vi "Preview HVAC.vi"(8 "error in (no error)":errorcluster, 11 "HVAC System Model in":refnum<class "HVAC System Model.lvclass">) -> (0 "error out":errorcluster, 3 "HVAC System Model out":refnum<class "HVAC System Model.lvclass">)   [LabVIEW 2013, in "HVAC System Model.lvlib" / "HVAC System Model.lvclass"]
uses:
  HVAC System Model.lvclass
  HVAC System Model.lvclass/HVAC System Model.ctl
  <vilib>/xml/Load XML File.vi
  <vilib>/xml/Close Reference(Node).vi
  Common/File IO/File IO.lvlib
  <vilib>/xml/NI_XML.lvlib
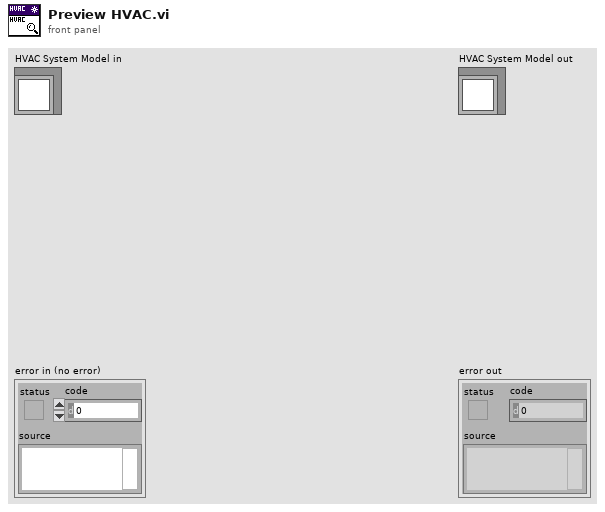
[diagram p1: front panel]
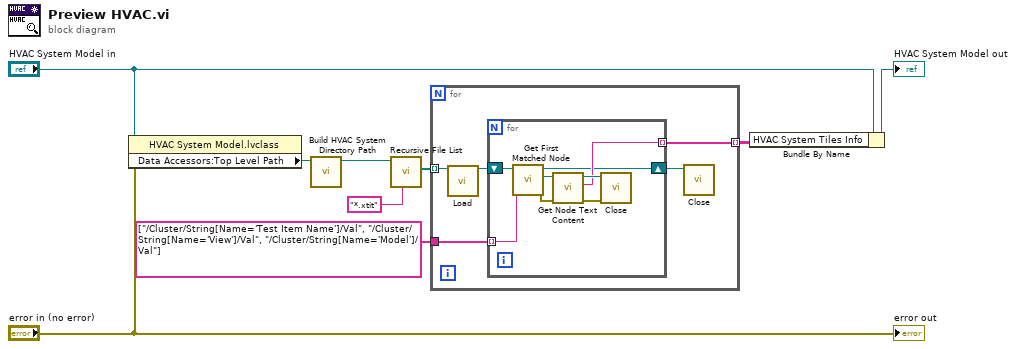
[diagram p0: block diagram]
diagram:
  n1 = property class="HVAC System Model.lvclass"(reference="HVAC System Model in", error in="error in (no error)") -> ("Data Accessors:Top Level Path"=w8:path)  [unwired: 2 out]
  n2 = call "Build HVAC System Directory Path.vi"("Top Level Path"=w8) -> ("HAVC System Directory Path"=w7:path)  [unwired: 10 in]
  n3 = call <vilib>:"Recursive File List.vi"("pattern"="*.xtit", "Folder Path"=w7) -> ("All Files in Dir"=w3:path[])  [unwired: 5 in, 4 out]
  n4 = for {
    tunnel: w3 -> [w12] mode=indexing
    tunnel: string[] ["/Cluster/String[Name='Test Item Name']/Val", "/Cluster/String[Name='View']/Val", "/Cluster/String[Name='Model']/Val"] -> [w13]
    tunnel: [w10] -> w2 mode=indexing
    n5 = call-poly <vilib>:"Load.vi"("path to XML document"=w12) -> ("DOM document out"=w14:refnum<k20>)  [unwired: 12 in, 2 out]
    n6 = for {
      shift-right: [w15] -> w11
      shift-left: w14 -> [w22]
      tunnel: w13 -> [w21] mode=indexing
      tunnel: [w18] -> w10 mode=indexing
      n7 = call <vilib>:"Get First Matched Node.vi"("XPath expression"=w21, "node in"=w22) -> ("error out"=w16:errorcluster, "node result"=w20:refnum<k20>, "node out"=w15:refnum<k20>)  [unwired: 7 in]
      n8 = call <vilib>:"Get Node Text Content.vi"("error in (no error)"=w16, "node in"=w20) -> ("error out"=w17:errorcluster, "node text"=w18:string, "node out"=w19:refnum<k20>)  [unwired: 7 in]
      n9 = call-poly <vilib>:"Close.vi"("error in (no error)"=w17, "node"=w19) -> ()  [unwired: 7 in, 1 out]
    }
    n10 = call-poly <vilib>:"Close.vi"("node"=w11) -> ()  [unwired: 8 in, 1 out]
  }
  n11 = Bundle By Name(cluster="HVAC System Model in", "HVAC System Tiles Info"=w2) -> (→"HVAC System Model out":refnum<class "HVAC System Model.lvclass">)
  "error out" <- "error in (no error)"
